vi "WILT Read File Paths Config File.vi"(8 "Error In":errorcluster, 9 "Config Data Input":string[](array[string]), 10 "General Configuration File Path":path, 11 "File Path Input":T1[](array[typedef])) -> (0 "Error Out":errorcluster, 3 "File Path Output":T1[](array[typedef]))   [LabVIEW 2016]
uses:
  Utility/Save File/File Setup (Public)/Type Definition/Save File DOE File Path Control.ctl
  Utility/Save File/File Setup (Public)/Type Definition/Save File DOE Data Save Filepaths.ctl
  <vilib>/Utility/error.llb/whitespace.ctl
  Utility/Type Definitions/UTILITY Default File Create.ctl
  Utility/Save File/Save File.lvlib
  Utility/Save File/File Setup.lvlib
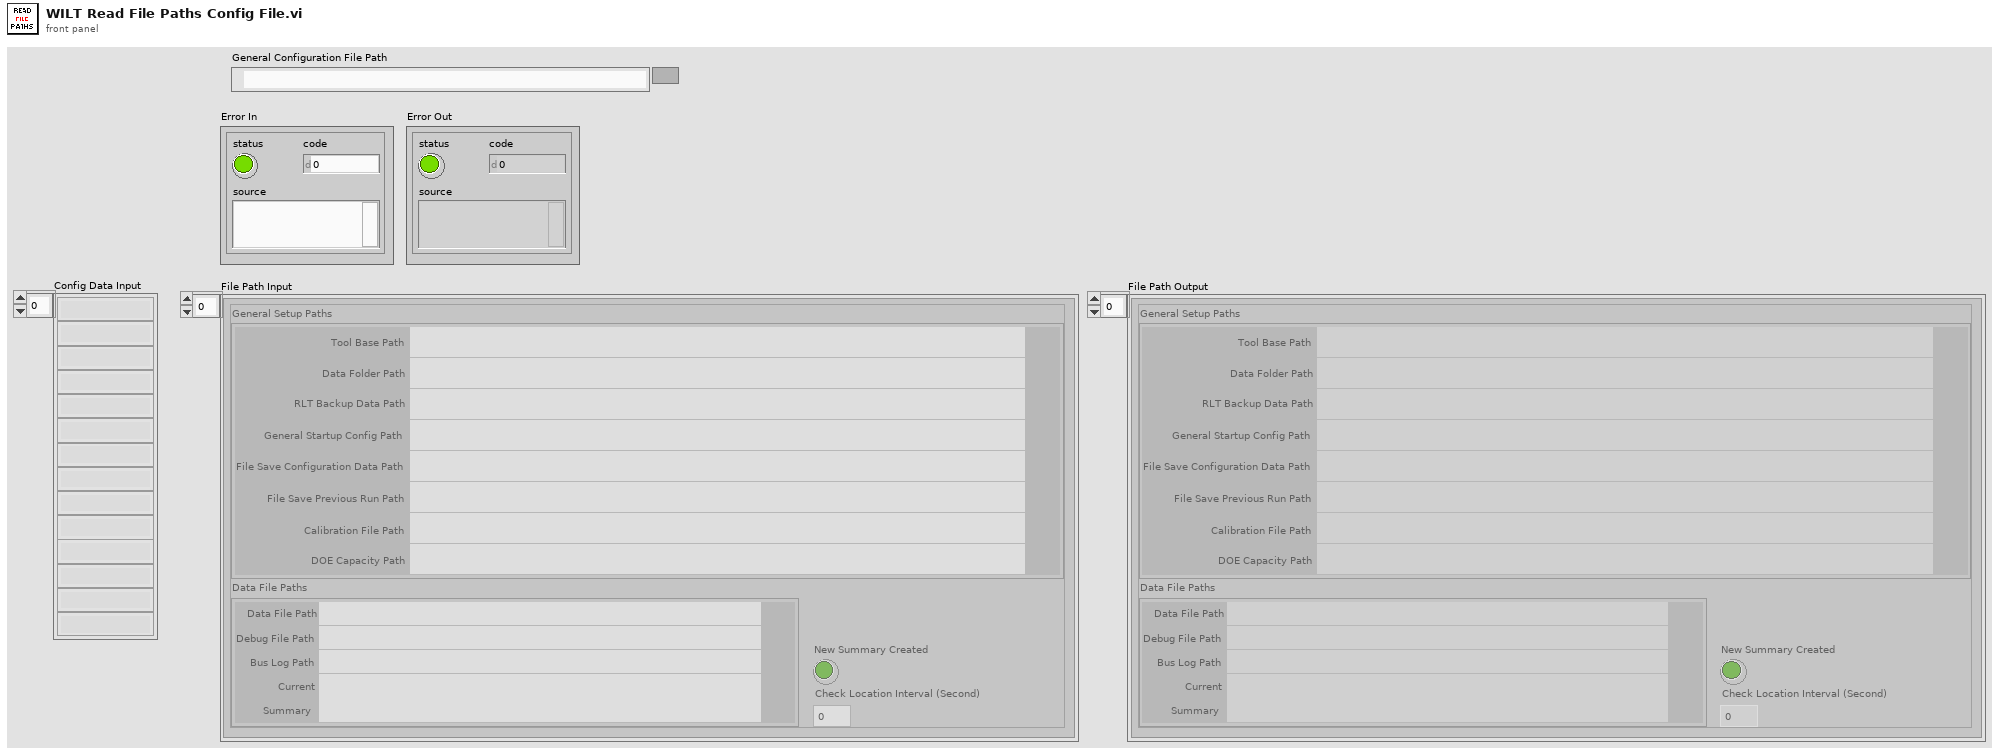
[diagram p1: front panel]
types:
  T1 = typedef "File Setup.lvlib/Save File DOE File Path Control.ctl" = cluster{"General Setup Paths":cluster{"Calibration File Path":path, "DOE Capacity Path":path, "Data Folder Path":path, "RLT Backup Data Path":path, "Tool Base Path":path, "General Startup Config Path":path, "File Save Previous Run Path":path, "File Save Configuration Data Path":path}, "Data File Paths":T2, "New Summary Created":bool, "Check Location Interval (Second)":i32}
  T2 = typedef "File Setup.lvlib/Save File DOE Data Save Filepaths.ctl" = cluster{"Data File Path":path, "Debug File Path":path, "Bus Log Path":path, "Current":path, "Summary":path}
  T3 = typedef "whitespace.ctl" = u16
  T4 = typedef "UTILITY Default File Create.ctl" = enum16{"Configuration File", "Debug Search File", "WILT Water Injection Times", "WILT Agilent Assignment", "WILT Save Status Path", "WILT General Config"}
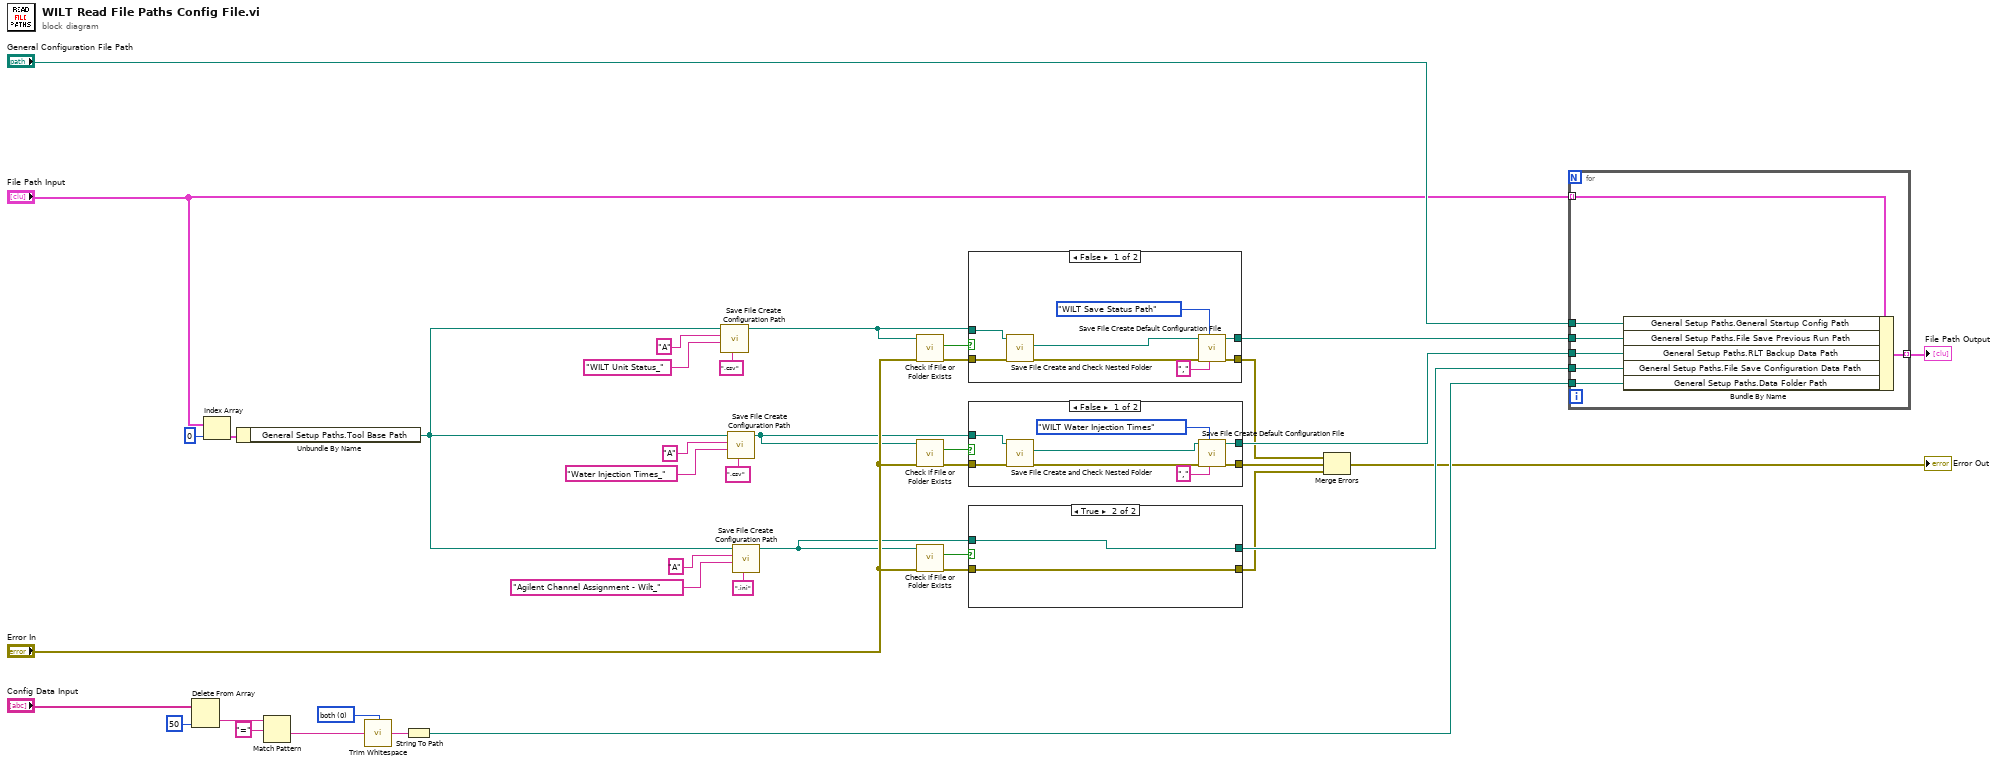
[diagram p0: block diagram]
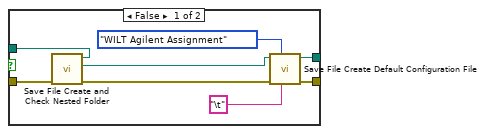
[diagram p2: hidden frame]
diagram:
  w38 = T3 0 items=["both", "start of string", "end of string"] ("location (both)")
  n1 = Delete From Array(array="Config Data Input", index=50) -> (deleted portion=w36:string)  [unwired: 1 in, 1 out]
  n2 = Index Array(array="File Path Input", index=0) -> (element=w14:T1)
  n3 = Unbundle By Name(w14) -> ("General Setup Paths.Tool Base Path"=w1:path)
  n4 = Match Pattern(string=w36, regular expression="=") -> (after substring=w37:string)  [unwired: 1 in, 3 out]
  n5 = call <vilib>:"Trim Whitespace.vi"("string"=w37, "location (both)"=w38) -> ("trimmed string"=w39:string)
  n6 = String To Path(string=w39) -> (path=w23:path)
  n7 = call "Save File Create Configuration Path.vi"("File Type (.ini)"=".csv", "Configuration Name"="WILT Unit Status_", "Station ID"="A", "Tool Base Path"=w1) -> ("New Configuration File Path"=w4:path)  [unwired: 6 in, 1 out]
  n8 = call "Save File Create Configuration Path.vi"("File Type (.ini)"=".csv", "Configuration Name"="Water Injection Times_", "Station ID"="A", "Tool Base Path"=w1) -> ("New Configuration File Path"=w3:path)  [unwired: 6 in, 1 out]
  n9 = call "Save File Create Configuration Path.vi"("File Type (.ini)"=".ini", "Configuration Name"="Agilent Channel Assignment - Wilt_", "Station ID"="A", "Tool Base Path"=w1) -> ("New Configuration File Path"=w2:path)  [unwired: 6 in, 1 out]
  n10 = call <vilib>:"Check if File or Folder Exists.vi"("error in (no error)"="Error In", "path"=w4) -> ("error out"=w31:errorcluster, "file or folder exists?"=w32:bool)  [unwired: 7 in, 1 out]
  n11 = call <vilib>:"Check if File or Folder Exists.vi"("error in (no error)"="Error In", "path"=w3) -> ("error out"=w29:errorcluster, "file or folder exists?"=w28:bool)  [unwired: 7 in, 1 out]
  n12 = call <vilib>:"Check if File or Folder Exists.vi"("error in (no error)"="Error In", "path"=w2) -> ("error out"=w25:errorcluster, "file or folder exists?"=w26:bool)  [unwired: 7 in, 1 out]
  n13 = case shown="False" w32 {
    tunnel: w4 -> [w48 w50]
    tunnel: [w45 w50] -> w30
    tunnel: w31 -> [w42 w49]
    tunnel: [w46 w49] -> w22
    frame False {
      n14 = call "Save File Create and Check Nested Folder.vi"("error in (no error)"=w42, "Extracted File Name"=w48) -> ("error out"=w47:errorcluster, "File Path"=w44:path)  [unwired: 7 in, 1 out]
      n15 = call "Save File Create Default Configuration File.vi"("delimiter (\\t)"="," ("delimiter (\\t)"), "Default File Create"=UTILITY_Default_File_Create."WILT Save Status Path", "Error In"=w47, "File Path In"=w44) -> ("Error Out"=w46:errorcluster, "File Path Out"=w45:path)  [unwired: 6 in]
    }
    frame True {
    }
  }
  n16 = case shown="False" w28 {
    tunnel: w3 -> [w58 w60]
    tunnel: [w55 w60] -> w27
    tunnel: w29 -> [w52 w59]
    tunnel: [w56 w59] -> w21
    frame False {
      n17 = call "Save File Create and Check Nested Folder.vi"("error in (no error)"=w52, "Extracted File Name"=w58) -> ("error out"=w57:errorcluster, "File Path"=w54:path)  [unwired: 7 in, 1 out]
      n18 = call "Save File Create Default Configuration File.vi"("delimiter (\\t)"="," ("delimiter (\\t)"), "Default File Create"=UTILITY_Default_File_Create."WILT Water Injection Times", "Error In"=w57, "File Path In"=w54) -> ("Error Out"=w56:errorcluster, "File Path Out"=w55:path)  [unwired: 6 in]
    }
    frame True {
    }
  }
  n19 = case shown="True" w26 {
    tunnel: w2 -> [w68 w70]
    tunnel: [w65 w70] -> w24
    tunnel: w25 -> [w62 w69]
    tunnel: [w66 w69] -> w20
    frame False {
      n20 = call "Save File Create and Check Nested Folder.vi"("error in (no error)"=w62, "Extracted File Name"=w68) -> ("error out"=w67:errorcluster, "File Path"=w64:path)  [unwired: 7 in, 1 out]
      n21 = call "Save File Create Default Configuration File.vi"("delimiter (\\t)"="\t" ("delimiter (\\t)"), "Default File Create"=UTILITY_Default_File_Create."WILT Agilent Assignment", "Error In"=w67, "File Path In"=w64) -> ("Error Out"=w66:errorcluster, "File Path Out"=w65:path)  [unwired: 6 in]
    }
    frame True {
    }
  }
  n22 = Merge Errors(w22, w21, w20) -> (→"Error Out":errorcluster)
  n23 = for {
    tunnel: "File Path Input" -> [w77] mode=indexing
    tunnel: w30 -> [w76]
    tunnel: w27 -> [w75]
    tunnel: w24 -> [w74]
    tunnel: w23 -> [w73]
    tunnel: [w72] -> w33 mode=indexing
    tunnel: "General Configuration File Path" -> [w71]
    n24 = Bundle By Name(cluster=w77, "General Setup Paths.General Startup Config Path"=w71, "General Setup Paths.File Save Previous Run Path"=w76, "General Setup Paths.RLT Backup Data Path"=w75, "General Setup Paths.File Save Configuration Data Path"=w74, "General Setup Paths.Data Folder Path"=w73) -> (w72:T1)
  }
  "File Path Output" <- w33
